vi "example test.vi"() -> (0 "input lookup error":errorcluster, 1 "init error":errorcluster, 2 "correct execution settings":bool, 3 "output lookup error":errorcluster, 4 "input error":errorcluster, 5 "serialization problem":errorcluster, 6 "no data written":bool, 7 "invalid configuration":errorcluster, 8 "final error":errorcluster, 9 "output error":errorcluster)   [LabVIEW 2014, in "SQLite tests.lvlib"]
doc: "This VI shows an example for how to test the Runtime functionality of the module. This will need to be modified according to module functionality."
uses:
  SQLite tests.lvlib
  module/configuration/SQLite configuration.lvclass
  <vilib>/NI/Tag Bus Module Framework/channel/channel classification.ctl
  <vilib>/NI/Tag Bus/tag/Data Type.ctl
  module/execution/SQLite runtime.lvclass
  <vilib>/NI/Tag Bus/dictionary/data dictionary.lvclass/data dictionary.ctl
  <vilib>/drjdpowell/SQLite Library/SQL Connection/Open (string).vi
  <vilib>/NI/Tag Bus/dictionary/lookup polymorphs/locate double.vi
  <vilib>/NI/Tag Bus/table/data polymorphs/write one/write Double.vi
  <vilib>/NI/Tag Bus/table/data polymorphs/read one/read Double.vi
  <vilib>/NI/Tag Bus/dictionary/search/find data index.vi
  <vilib>/NI/Tag Bus/dictionary/search/search string list.vi
  <vilib>/NI/Tag Bus/dictionary/tag not found.vi
  <vilib>/drjdpowell/SQLite Library/SQL Connection/Connection.lvclass
  <vilib>/NI/Tag Bus/dictionary/data dictionary.lvclass
  <vilib>/NI/Tag Bus/table/data table.lvlib
  <vilib>/NI/Tag Bus Module Framework/channel/TBM channel.lvclass
  <vilib>/NI/Tag Bus/tag/tag descriptor.lvclass
  <vilib>/NI/Configuration Framework/serializable configuration/NISE_CEF_serializable configuration.lvclass
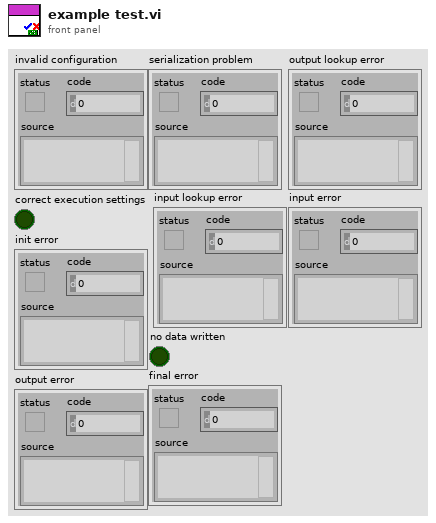
[diagram p1: front panel]
types:
  T1 = enum16{"New or existing", "Existing", "Read only"}
  T2 = typedef "TBM channel.lvclass/channel classification.ctl" = enum16{"input data", "output data", "processing parameter", "processing result"}
  T3 = typedef "tag bus.lvlib/tag descriptor.lvclass/Data Type.ctl" = enum16{"Double", "Single", "I64", "I32", "I16", "I8", "U64", "U32", "U16", "U8", "Boolean", "String", "Array of Double", "Array of Single", "Array of I64", "Array of I32", "Array of I16", "Array of I8", "Array of U64", "Array of U32", "Array of U16", "Array of U8", "Array of Boolean", "Array of String"}
  T4 = cluster{"channel":refnum<class "TBM channel.lvclass">}
  T5 = typedef "TBM channel.lvclass/data tables.ctl" = cluster{"input data":T6, "processing parameter":T6, "processing result":T6, "output data":T6}
  T6 = typedef "tag bus.lvlib/dictionary table pair.ctl" = cluster{"data dictionary":refnum<class "data dictionary.lvclass">, "data table":T7}
  T7 = typedef "tag bus.lvlib/data table.lvlib/data table.ctl" = cluster{"Double":dbl[], "Single":sgl[], "I64":i64[], "I32":i32[], "I16":i16[], "I8":i8[], "U64":u64[], "U32":u32[], "U16":u16[], "U8":u8[], "Boolean":bool[], "String":string[], "Array of Double":cluster{"DBL Array":dbl[]}[], "Array of Single":cluster{"SGL Array":sgl[]}[], "Array of I64":cluster{"I64 Array":i64[]}[], "Array of I32":cluster{"I32 Array":i32[]}[], "Array of I16":cluster{"I16 Array":i16[]}[], "Array of I8":cluster{"I8 Array":i8[]}[], "Array of U64":cluster{"U64 Array":u64[]}[], "Array of U32":cluster{"U32 Array":u32[]}[], "Array of U16":cluster{"U16 Array":u16[]}[], "Array of U8":cluster{"U8 Array":u8[]}[], "Array of Boolean":cluster{"Boolean Array":bool[]}[], "Array of String":cluster{"String Array":string[]}[]}
  T8 = typedef "TBM module execution interface.lvclass/execution settings.ctl" = cluster{"reads inputs":bool, "processes data":bool, "writes outputs":bool}
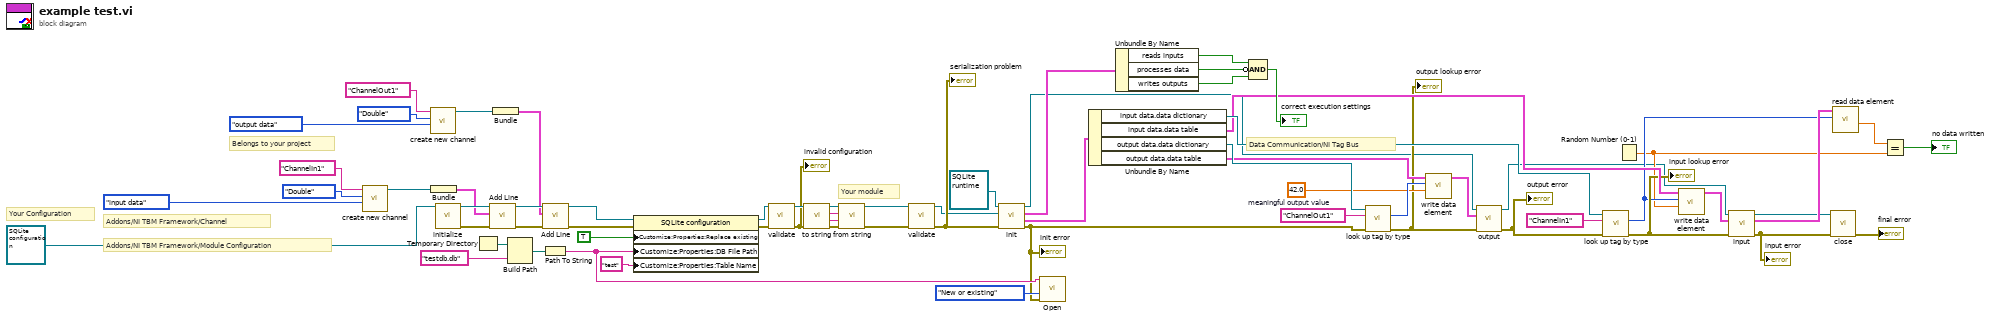
[diagram p0: block diagram]
diagram:
  w30 = 42.0  # meaningful output value
  # "Data Communication/NI Tag Bus"
  # "Your module"
  # "Your Configuration"
  # "Addons/NI TBM Framework/Module Configuration"
  # "Belongs to your project"
  # "Addons/NI TBM Framework/Channel"
  n1 = call <vilib>:"create new channel.vi"("channel classification"=channel_classification."input data", "data type"=Data_Type."Double", "channel name"="ChannelIn1") -> ("channel"=w21:refnum<class "TBM channel.lvclass">)  [unwired: 8 in]
  n2 = call <vilib>:"create new channel.vi"("channel classification"=channel_classification."output data", "data type"=Data_Type."Double", "channel name"="ChannelOut1") -> ("channel"=w19:refnum<class "TBM channel.lvclass">)  [unwired: 8 in]
  n3 = Bundle("channel"=w21) -> (w20:T4)  [unwired: 1 in]
  n4 = call <vilib>:"initialize.vi"("configuration in"=refnum<class "SQLite configuration.lvclass"> refnum ("tag bus configurable plugin module configuration")) -> ("error out"=w22:errorcluster, "configuration out"=w23:refnum<class "SQLite configuration.lvclass">)  [unwired: 8 in, 1 out]
  n5 = Temporary Directory() -> (w15:path)
  n6 = call "Add Line.vi"("error in"=w22, "Line"=w20, "SQLite configuration in"=w23) -> ("error out"=w24:errorcluster, "SQLite configuration out"=w25:refnum<class "SQLite configuration.lvclass">)  [unwired: 6 in, 1 out]
  n7 = Bundle("channel"=w19) -> (w18:T4)  [unwired: 1 in]
  n8 = Build Path(base path=w15, name or relative path="testdb.db") -> (appended path=w12:path)
  n9 = Path To String(path=w12) -> (string=w3:string)
  n10 = call "Add Line.vi"("error in"=w24, "Line"=w18, "SQLite configuration in"=w25) -> ("error out"=w10:errorcluster, "SQLite configuration out"=w17:refnum<class "SQLite configuration.lvclass">)  [unwired: 6 in, 1 out]
  n11 = property class="SQLite configuration"(reference=w17, error in=w10, "Customize:Properties:Replace existing"=TRUE ("Replace existing"), "Customize:Properties:DB File Path"=w3, "Customize:Properties:Table Name"="test" ("Table Name")) -> (reference out=w11:refnum<class "SQLite configuration.lvclass">, error out=w9:errorcluster)
  n12 = call-dynamic "validate.vi"("error in"=w9, "SQLite configuration in"=w11) -> ("error out"=w60:errorcluster, "SQLite configuration out"=w61:refnum<class "SQLite configuration.lvclass">)  [unwired: 8 in]
  "invalid configuration" <- w60
  n13 = call-dynamic "to string.vi"("error in"=w60, "SQLite configuration in"=w61) -> ("error out"=w56:errorcluster, "data"=w57:string, "version"=w58:string, "SQLite configuration out"=w59:refnum<class "SQLite configuration.lvclass">)  [unwired: 6 in]
  n14 = call-dynamic "from string.vi"("error in"=w56, "data"=w57, "version"=w58, "SQLite configuration in"=w59) -> ("error out"=w54:errorcluster, "SQLite configuration out"=w55:refnum<class "SQLite configuration.lvclass">)  [unwired: 6 in]
  n15 = call-dynamic "validate.vi"("error in"=w54, "SQLite configuration in"=w55) -> ("error out"=w52:errorcluster, "SQLite configuration out"=w51:refnum<class "SQLite configuration.lvclass">)  [unwired: 8 in]
  "serialization problem" <- w52
  n16 = call-dynamic "init.vi"("error in"=w52, "TBM module configuration in"=w51, "SQLite runtime in"=refnum<class "SQLite runtime.lvclass"> refnum ("tag bus configurable plugin module")) -> ("error out"=w1:errorcluster, "data allocations"=w45:T5, "execution settings"=w50:T8, "SQLite runtime out"=w8:refnum<class "SQLite runtime.lvclass">)  [unwired: 5 in]
  "init error" <- w1
  n17 = call-poly <vilib>:"Open.vi"("error in (no error)"=w1, "File Option"=T1."New or existing", "db file"=w3) -> ()  [unwired: 7 in, 2 out]
  n18 = Unbundle By Name(w45) -> ("input data.data dictionary"=w44:refnum<class "data dictionary.lvclass">, "input data.data table"=w42:T7, "output data.data dictionary"=w34:refnum<class "data dictionary.lvclass">, "output data.data table"=w31:T7)
  n19 = Unbundle By Name(w50) -> ("reads inputs"=w47:bool, "processes data"=w49:bool, "writes outputs"=w48:bool)
  n20 = Compound Arithmetic op=AND(w47, invert w49, w48) -> (→"correct execution settings":bool)
  n21 = call-poly <vilib>:"look up tag by type.vi"("error in"=w1, "name"="ChannelOut1" ("channel name"), "data dictionary in"=w34) -> ("error out"=w29:errorcluster, "index"=w32:i32)  [unwired: 6 in, 1 out]
  "output lookup error" <- w29
  n22 = call-poly <vilib>:"write data element.vi"("value"=w30, "index"=w32, "data table in"=w31) -> ("data table out"=w28:T7)  [unwired: 8 in]
  n23 = call-dynamic "output.vi"("error in"=w29, "data table in"=w28, "SQLite runtime in"=w8) -> ("error out"=w4:errorcluster, "SQLite runtime out"=w7:refnum<class "SQLite runtime.lvclass">)  [unwired: 6 in, 1 out]
  "output error" <- w4
  n24 = call-poly <vilib>:"look up tag by type.vi"("error in"=w4, "name"="ChannelIn1" ("channel name"), "data dictionary in"=w44) -> ("error out"=w41:errorcluster, "index"=w38:i32)  [unwired: 6 in, 1 out]
  "input lookup error" <- w41
  n25 = Random Number (0-1)() -> (number: 0 to 1=w37:dbl)
  n26 = call-poly <vilib>:"write data element.vi"("value"=w37, "index"=w38, "data table in"=w42) -> ("data table out"=w40:T7)  [unwired: 8 in]
  n27 = call-dynamic "input.vi"("error in"=w41, "data table in"=w40, "SQLite runtime in"=w7) -> ("error out"=w5:errorcluster, "data table out"=w39:T7, "SQLite runtime out"=w6:refnum<class "SQLite runtime.lvclass">)  [unwired: 6 in]
  "input error" <- w5
  n28 = call-dynamic "close.vi"("error in"=w5, "SQLite runtime in"=w6) -> ("error out"=→"final error":errorcluster)  [unwired: 9 in]
  n29 = call-poly <vilib>:"read data element.vi"("index"=w38, "data table in"=w39) -> ("value"=w36:dbl)  [unwired: 8 in, 1 out]
  n30 = Equal?(x=w36, y=w37) -> (x = y?=→"no data written":bool)
